vi "3DAvg.vi"(1 "3D In":dbl[][][](array[numeric])) -> (0 "2D Out":dbl[][](array[numeric]))   [LabVIEW 2015]
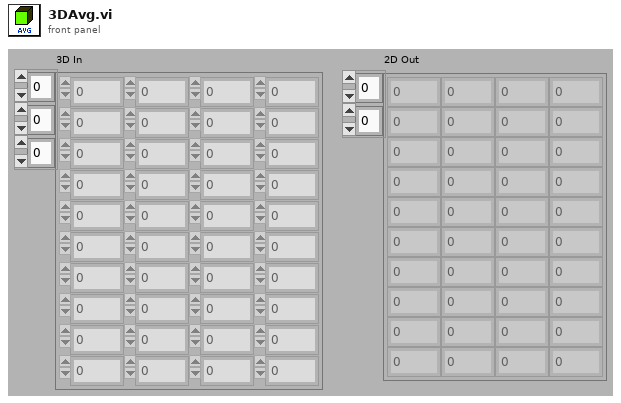
[diagram p1: front panel]
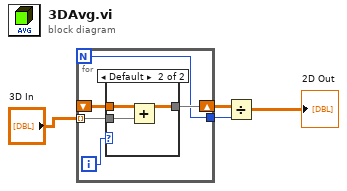
[diagram p0: block diagram]
diagram:
  n1 = for {
    N -> [w5]
    tunnel: "3D In" -> [w7] mode=indexing
    shift-right: [w9] -> w4
    shift-left: _ -> [w8]
    tunnel: [w5] -> w3
    i -> [w6]
    n2 = case shown="Default" w6 {
      tunnel: [w10 w13] -> w9
      tunnel: w8 -> [_ w12]
      tunnel: w7 -> [w10 w11]
      frame 0 {
      }
      frame Default {
        n3 = Add(x=w12, y=w11) -> (x+y=w13:dbl[][])
      }
    }
  }
  n4 = Divide(x=w4, y=w3) -> (x/y=→"2D Out":dbl[][])
